vi "Actor Core.vi"(8 "error in":errorcluster, 11 "WS Test Client in":refnum<class "WS Test Client.lvclass">) -> (0 "error out":errorcluster, 3 "Actor out":refnum<class "Actor.lvclass">)   [LabVIEW 2016, in "Echo Broadcast Test Without Server Manager.lvlib" / "WS Test Client.lvclass"]
doc: "(<B>Filename</B>: Actor Framework.lvlib:Actor.lvclass:Actor Core.vi)\n\nReceives messages to the actor, reacts to them, and initiates any error handling that may shut the actor down.\n\nDescendant classes may override this VI to append parallel tasks for the actor to complete while it handles messages. Overrides use the Call Parent Method node."
uses:
  WS Test Client.lvclass
  C:/Program Files (x86)/National Instruments/LabVIEW 2016/vi.lib/ActorFramework/Actor/Actor.lvclass
  <vilib>/ActorFramework/Actor/Actor.lvclass
  <vilib>/ActorFramework/Message Enqueuer/Message Enqueuer.lvclass
  WS Test Client.lvclass/WS Test Client.ctl
  <vilib>/ActorFramework/Actor/Actor.lvclass/Actor.ctl
  <vilib>/ActorFramework/Message Enqueuer/Message Enqueuer.lvclass/Message Enqueuer.ctl
  <vilib>/ActorFramework/Message Enqueuer/Init from Existing Queue.vi
  <vilib>/ActorFramework/Message Enqueuer/Enqueue.vi
  <vilib>/ActorFramework/Stop Msg/Stop Msg.lvclass
  C:/Program Files (x86)/National Instruments/LabVIEW 2016/vi.lib/ActorFramework/Message/Message.lvclass
  <vilib>/ActorFramework/Message Priority Queue/Priority Enqueue.vi
  <vilib>/MGI/Monitored Actor/Monitored Actor/Monitored Actor/Monitored Actor.lvclass
  WebSocket Actor/WebSocket Connection Messages/Send to Peer Msg/Send to Peer Msg.lvclass
panel:
  in  "Send":bool
  in  "Data To Send":string
  in  "Exit":bool
  out "Echoed Data":string
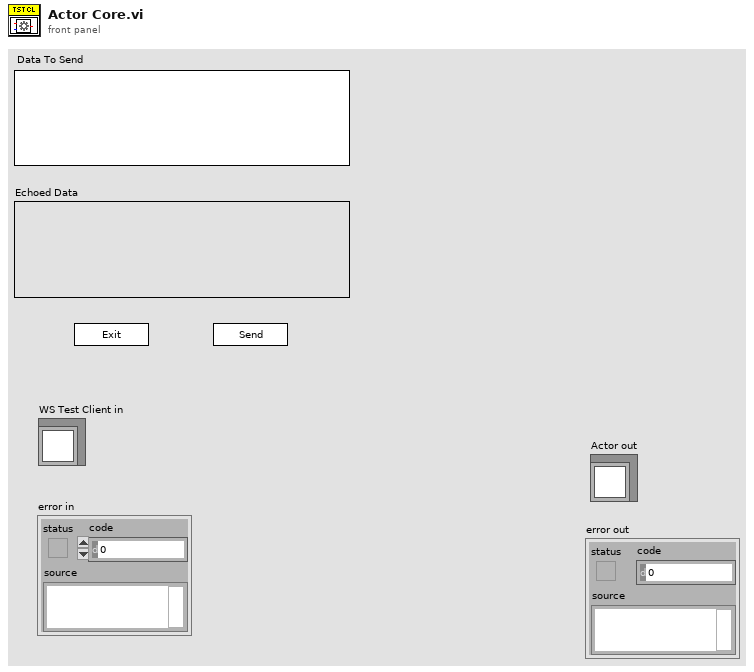
[diagram p1: front panel]
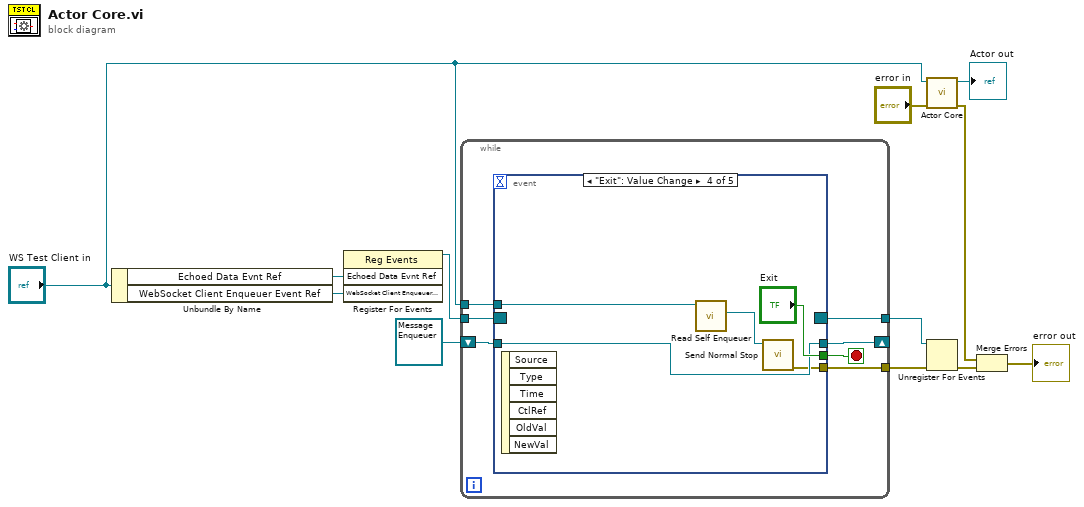
[diagram p0: block diagram]
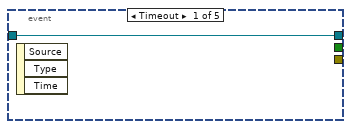
[diagram p2: hidden frame]
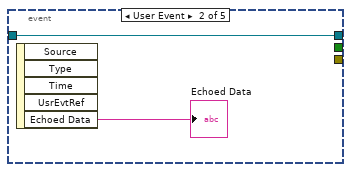
[diagram p3: hidden frame]
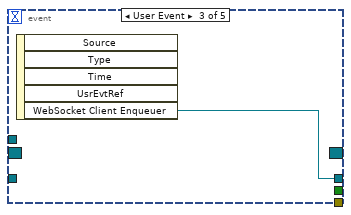
[diagram p4: hidden frame]
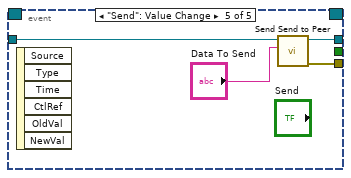
[diagram p5: hidden frame]
diagram:
  n1 = Unbundle By Name("WS Test Client in") -> ("Echoed Data Evnt Ref"=w9:refnum<user-event>, "WebSocket Client Enqueuer Event Ref"=w7:refnum<user-event>)
  n2 = register-events(w9, w7) -> (reference out=w8:refnum<event-registration>)  [unwired: 2 in, 1 out]
  n3 = while {
    tunnel: w8 -> [w19]
    shift-right: [w17] -> _
    shift-left: refnum<class "Message Enqueuer.lvclass"> refnum ("WebSocket Client Enqueuer") -> [w16]
    tunnel: [w15] -> w5
    tunnel: "WS Test Client in" -> [w14]
    tunnel: [w13] -> w1
    stop <- w18 stop-if-true
    n4 = event shown="[3] \"Exit\": Value Change" {
      selector: w19 -> [_ _ _ _ _]
      dyn-events: [_ _ _ _ _] -> w15
      timeout: _ -> [_ _ _ _ _]
      tunnel: [_ _ _ "Exit" _] -> w18
      tunnel: [w20 w21 w23 w27 w30] -> w17
      tunnel: w16 -> [w20 w21 _ w27 w31]
      tunnel: w14 -> [_ _ _ w26 _]
      tunnel: [_ _ _ w24 w29] -> w13
      event Timeout {
        n5 = event-data() -> ()  [unwired: 1 in, 3 out]
      }
      event User Event {
        n6 = event-data() -> ("Echoed Data"=→"Echoed Data":string)  [unwired: 1 in, 4 out]
      }
      event User Event {
        n7 = event-data() -> ("WebSocket Client Enqueuer"=w23:refnum<class "Message Enqueuer.lvclass">)  [unwired: 1 in, 4 out]
      }
      event "Exit": Value Change {
        n8 = event-data() -> ()  [unwired: 1 in, 6 out]
        n9 = call <vilib>:"Read Self Enqueuer.vi"("Actor"=w26) -> ("Self Enqueuer"=w25:refnum<class "Message Enqueuer.lvclass">)  [unwired: 10 in]
        n10 = call <vilib>:"Send Normal Stop.vi"("Message Enqueuer"=w25) -> ("error out"=w24:errorcluster)  [unwired: 10 in]
      }
      event "Send": Value Change {
        n11 = event-data() -> ()  [unwired: 1 in, 6 out]
        n12 = call "Send Send to Peer.vi"("Data"="Data To Send", "Message Enqueuer in"=w31) -> ("error out"=w29:errorcluster, "Message Enqueuer out"=w30:refnum<class "Message Enqueuer.lvclass">)  [unwired: 8 in]
      }
    }
  }
  n13 = call-parent "Actor Core.vi"("error in"="error in", "Actor in"="WS Test Client in") -> ("error out"=w12:errorcluster, "Actor out"=→"Actor out":refnum<class "Actor.lvclass">)  [unwired: 8 in]
  n14 = Unregister For Events(event registration refnum=w5, error in=w1) -> (error out=w3:errorcluster)
  n15 = Merge Errors(w12, w3) -> (→"error out":errorcluster)
